vi "EPTx Basic Example FPGA test.vi"() -> ()   [LabVIEW 2019]
uses:
  <vilib>/Powertrain Controls/Device Drivers/Engine Position Tracking/EPTx/RevA/FPGA/Controls/EPTxTooth.ctl
  <vilib>/Powertrain Controls/Device Drivers/Engine Position Tracking/EPTx/RevA/FPGA/Controls/EPTxConfig.ctl
  <vilib>/Powertrain Controls/Device Drivers/Engine Position Tracking/EPTx/RevA/FPGA/Controls/EPTxSupervisor.ctl
  <vilib>/Platform/TimedLoop/XDataNode/timing_clust.ctl
  <vilib>/Platform/TimedLoop/XDataNode/nitl_modes.ctl
  <vilib>/Platform/TimedLoop/XDataNode/wakeup.ctl
  <vilib>/Powertrain Controls/Device Drivers/Engine Position Tracking/EPTx/RevA/FPGA/Controls/EPTxAAPControl.ctl
  <vilib>/Powertrain Controls/Device Drivers/Engine Position Tracking/EPTx/RevA/FPGA/Controls/EPTxSignals.ctl
  <vilib>/Powertrain Controls/Device Drivers/Engine Position Tracking/EPTx/RevA/FPGA/Controls/EPTxControl.ctl
  <vilib>/rvi/Emulation/niFpgaGetClockAttributes.vi
  <vilib>/rvi/Emulation/niFpgaSctlEmulationGetInTimedLoop.vi
  <vilib>/rvi/Emulation/niFpgaEmulationReportErrorSimple.vi
  <vilib>/rvi/eio/common/nirviEmuTemplateMethod_errors.vi
  <vilib>/rvi/Emulation/niFpgaCriticalErrorInLSC.vi
  <vilib>/eio/EIONode/EIONode.xnode
  <vilib>/Platform/TimedLoop/XDataNode/XDataNode.xnode
  <vilib>/Platform/TimedLoop/XDataNode/XDNodeRunTimeDep.lvlib
  <vilib>/Powertrain Controls/Device Drivers/Engine Position Tracking/EPTx/RevA/FPGA/EPTx - RevA - FPGA.lvlib
panel:
  in  "Watchdog":bool
  in  "Sim Rate":fxp<+,24,6> format="%.20g"
  in  "Sim Enable":bool
  in  "Clear Errors":bool
  in  "Sync Enable":bool
  out "Watchdog Error":bool
  out "Aux Warning":bool
  out "Pattern Error":bool
  out "Ratio Error":bool
  out "Overflow":bool
  out "Stall":bool
  out "Rcvg Primary":bool
  out "Config":bool
  out "AvgSpeed":fxp<+,17,15> format="%.7g"
  out "CADRate":fxp<+,22,8> format="%.17g"
  out "HistoryCAD":fxp<+,11,11>
  out "MaxCAD":fxp<+,11,11>
  out "CurrentCAD":fxp<+,18,11> format="%.11g"
  out "Sync":bool
  in  "Cylinder1_L_F [CAD]":fxp<+,18,11> format="%.11g"
  in  "Cylinder1_L_R [CAD]":fxp<+,18,11> format="%.11g"
  in  "Cylinder1_H_F [CAD]":fxp<+,18,11> format="%.11g"
  in  "Cylinder1_H_R [CAD]":fxp<+,18,11> format="%.11g"
  in  "FallingCAD":fxp<+,18,11> format="%.11g"
  in  "RisingCAD":fxp<+,18,11> format="%.11g"
  in  "Enable":bool
  in  "当前转速":fxp<+,24,14>
  out "EPTxSupervisor":T1
  in  "EPTxConfig":T2
  out "EPTxTooth":T3
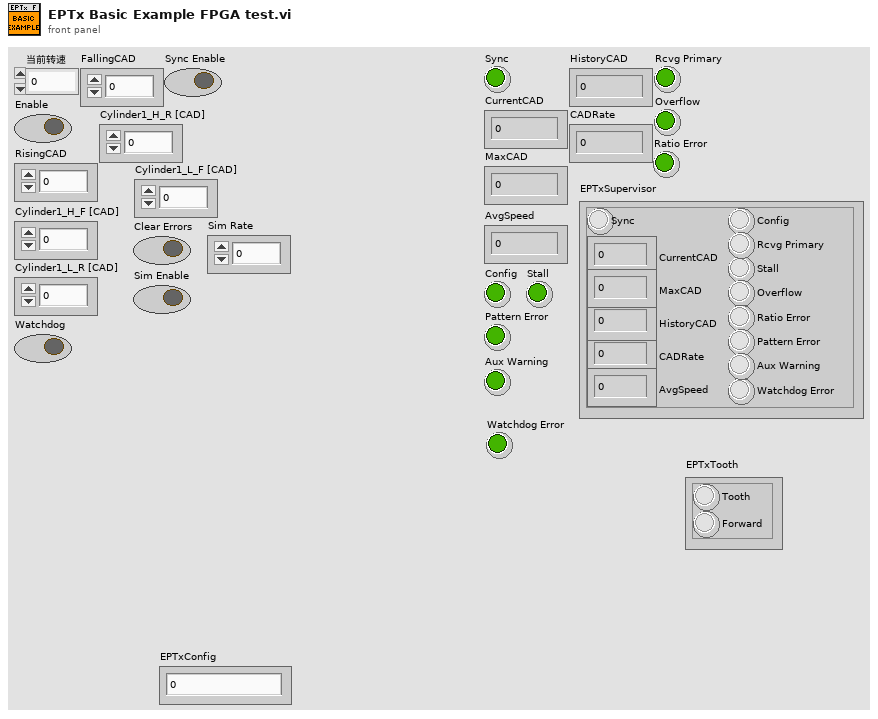
[diagram p1: front panel]
types:
  T1 = typedef "EPTx - RevA - FPGA.lvlib/EPTxSupervisor.ctl" = cluster{"Sync":bool, "CurrentCAD":fxp<+,18,11>, "MaxCAD":fxp<+,11,11>, "HistoryCAD":fxp<+,11,11>, "CADRate":fxp<+,22,8>, "AvgSpeed":fxp<+,17,15>, "Config":bool, "Rcvg Primary":bool, "Stall":bool, "Overflow":bool, "Ratio Error":bool, "Pattern Error":bool, "Aux Warning":bool, "Watchdog Error":bool}
  T2 = typedef "EPTx - RevA - FPGA.lvlib/EPTxConfig.ctl" = u64
  T3 = typedef "EPTx - RevA - FPGA.lvlib/EPTxTooth.ctl" = cluster{"Tooth":bool, "Forward":bool}
  T4 = typedef "XDNodeRunTimeDep.lvlib/timing_clust.ctl" = cluster{"Expected End [f-1]":u64, "Actual End [f-1]":u64, "Finished Late? [f-1]":bool, "Expected End [i-1]":u64, "Actual End [i-1]":u64, "Finished Late? [i-1]":bool, "Expected Start [i]":u64, "Actual Start [i]":u64, "Expected Start [f]":u64, "Actual Start [f]":u64, "Source Name":string, "Structure Name":string, "Period":i64, "Deadline":i64, "Offset":i64, "Start":i64, "Priority":i32, "Timeout":i32, "Mode":T5, "Wakeup Reason":T6, "Error":errorcluster, "Source Type":string, "Secondary Source Type":string, "Global End Time":u64, "Global Start Time":u64, "Frame Duration":u64, "Iteration Duration":u64, "Assigned CPU":i32, "I/O Scan Engine Mode":u32}
  T5 = typedef "XDNodeRunTimeDep.lvlib/nitl_modes.ctl" = enum32{"No Change", "Process missed periods, maintain original phase", "Discard missed periods, maintain original phase", "Process missed periods, ignore original phase", "Discard missed periods, ignore original phase"}
  T6 = typedef "XDNodeRunTimeDep.lvlib/wakeup.ctl" = enum32{"Normal", "Aborted", "Asynchronous wakeup", "Timing source error", "Timed loop error", "Timeout"}
  T7 = typedef "EPTx - RevA - FPGA.lvlib/EPTxControl.ctl" = cluster{"Sync Enable":bool, "Clear Errors":bool, "Sim Enable":bool, "Sim Rate":fxp<+,24,6>, "Watchdog":bool}
  T8 = cluster{"Cylinder1_H_R [CAD]":fxp<+,18,11>, "Cylinder1_H_F [CAD]":fxp<+,18,11>, "Cylinder1_L_R [CAD]":fxp<+,18,11>, "Cylinder1_L_F [CAD]":fxp<+,18,11>}
  T9 = typedef "EPTx - RevA - FPGA.lvlib/EPTxAAPControl.ctl" = cluster{"Enable":bool, "RisingCAD":fxp<+,18,11>, "FallingCAD":fxp<+,18,11>}
  T10 = typedef "EPTx - RevA - FPGA.lvlib/EPTxSignals.ctl" = cluster{"Primary":bool, "Aux 1":bool, "Aux 2":bool, "Aux 3":bool, "Aux 4":bool}
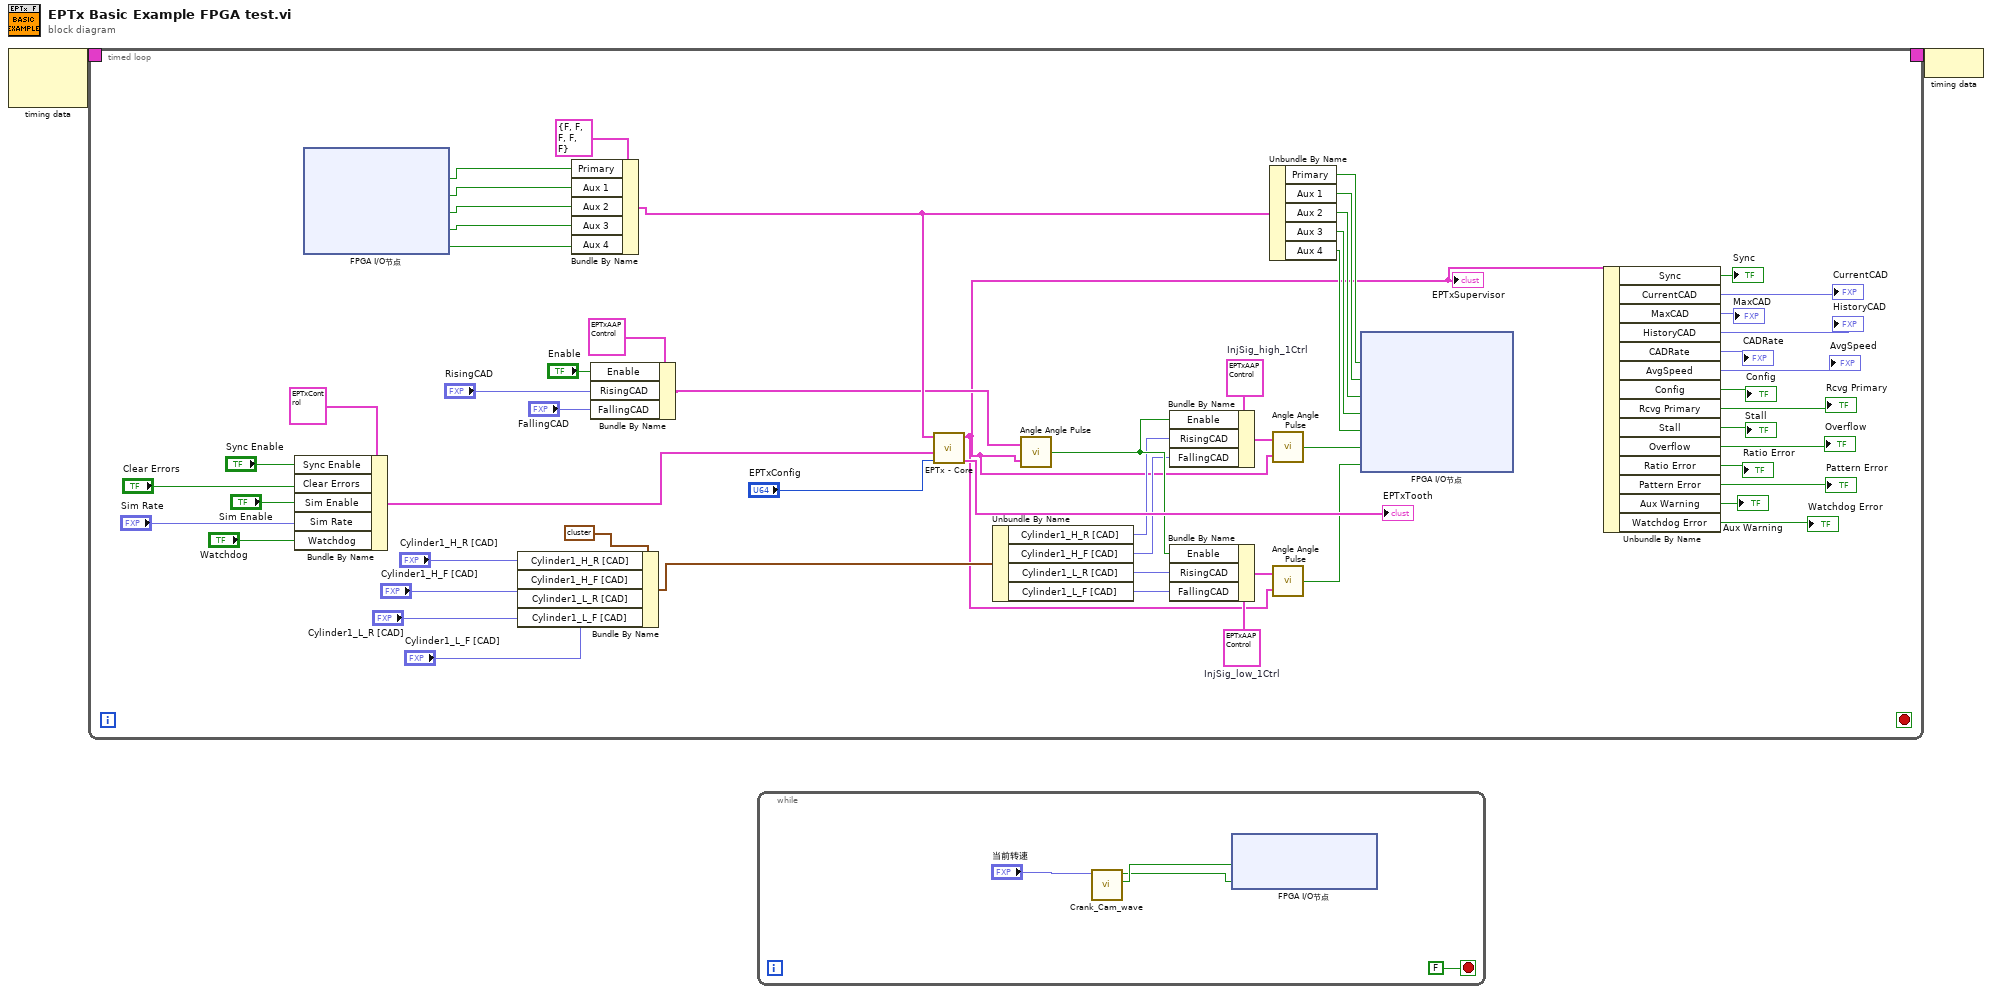
[diagram p0: block diagram]
diagram:
  n1 = node-c288() -> (w2:T4)  [unwired: 2 in]
  n2 = timed-loop {
    timing: w2 -> [_]
    timing-out: [_] -> w1
    stop <- _ stop-if-true
    w51 = T9 {"Enable"=FALSE, "RisingCAD"=0.0, "FallingCAD"=0.0}  # InjSig_low_1Ctrl
    w52 = T9 {"Enable"=FALSE, "RisingCAD"=0.0, "FallingCAD"=0.0}  # InjSig_high_1Ctrl
    n3 = Bundle By Name(cluster=T7 {"Sync Enable"=FALSE, "Clear Errors"=FALSE, "Sim Enable"=FALSE, "Sim Rate"=0.0, "Watchdog"=FALSE} ("EPTxControl"), "Sync Enable"="Sync Enable", "Clear Errors"="Clear Errors", "Sim Enable"="Sim Enable", "Sim Rate"="Sim Rate", "Watchdog"="Watchdog") -> (w3:T7)
    n4 = xnode "FPGA I/O节点"() -> ("Connector1/DIO0"=w40:bool, "Connector1/DIO1"=w39:bool, "Connector1/DIO2"=w38:bool, "Connector1/DIO3"=w37:bool, "Connector1/DIO4"=w36:bool)  [unwired: 5 in, 5 out]
    n5 = Bundle By Name(cluster=T8 {"Cylinder1_H_R [CAD]"=0.0, "Cylinder1_H_F [CAD]"=0.0, "Cylinder1_L_R [CAD]"=0.0, "Cylinder1_L_F [CAD]"=0.0} ("CylinderSig_1"), "Cylinder1_H_R [CAD]"="Cylinder1_H_R [CAD]", "Cylinder1_H_F [CAD]"="Cylinder1_H_F [CAD]", "Cylinder1_L_R [CAD]"="Cylinder1_L_R [CAD]", "Cylinder1_L_F [CAD]"="Cylinder1_L_F [CAD]") -> (w25:T8)
    n6 = Bundle By Name(cluster=T10 {"Primary"=FALSE, "Aux 1"=FALSE, "Aux 2"=FALSE, "Aux 3"=FALSE, "Aux 4"=FALSE} ("EPTxSignals"), "Primary"=w40, "Aux 1"=w39, "Aux 2"=w38, "Aux 3"=w37, "Aux 4"=w36) -> (w41:T10)
    n7 = Bundle By Name(cluster=T9 {"Enable"=FALSE, "RisingCAD"=0.0, "FallingCAD"=0.0} ("AAPControl_1str"), "Enable"="Enable", "RisingCAD"="RisingCAD", "FallingCAD"="FallingCAD") -> (w31:T9)
    n8 = call <vilib>:"EPTx - Core.vi"("EPTxConfig"="EPTxConfig", "EPTxControl"=w3, "EPTxSignals"=w41) -> ("EPTxTooth"=→"EPTxTooth":T3, "EPTxSupervisor"=w24:T1)  [unwired: 7 in]
    "EPTxSupervisor" <- w24
    n9 = Unbundle By Name(w25) -> ("Cylinder1_H_R [CAD]"=w48:fxp<+,18,11>, "Cylinder1_H_F [CAD]"=w47:fxp<+,18,11>, "Cylinder1_L_R [CAD]"=w46:fxp<+,18,11>, "Cylinder1_L_F [CAD]"=w45:fxp<+,18,11>)
    n10 = call <vilib>:"Angle Angle Pulse.vi"("EPTxSupervisor"=w24, "AAPControl"=w31) -> ("AAP"=w49:bool)
    n11 = Bundle By Name(cluster=w52, "Enable"=w49, "RisingCAD"=w48, "FallingCAD"=w47) -> (w53:T9)
    n12 = Bundle By Name(cluster=w51, "Enable"=w49, "RisingCAD"=w46, "FallingCAD"=w45) -> (w50:T9)
    n13 = Unbundle By Name(w41) -> ("Primary"=w58:bool, "Aux 1"=w57:bool, "Aux 2"=w56:bool, "Aux 3"=w55:bool, "Aux 4"=w54:bool)
    n14 = call <vilib>:"Angle Angle Pulse.vi"("EPTxSupervisor"=w24, "AAPControl"=w53) -> ("AAP"=w44:bool)
    n15 = call <vilib>:"Angle Angle Pulse.vi"("EPTxSupervisor"=w24, "AAPControl"=w50) -> ("AAP"=w43:bool)
    n16 = xnode "FPGA I/O节点"("Connector0/DIO4"=w58, "Connector0/DIO5"=w57, "Connector0/DIO6"=w56, "Connector0/DIO7"=w55, "Connector0/DIO8"=w54, "Connector0/DIO9"=w44, "Connector0/DIO10"=w43) -> ()  [unwired: 7 in, 7 out]
    n17 = Unbundle By Name(w24) -> ("Sync"=→"Sync":bool, "CurrentCAD"=→"CurrentCAD":fxp<+,18,11>, "MaxCAD"=→"MaxCAD":fxp<+,11,11>, "HistoryCAD"=→"HistoryCAD":fxp<+,11,11>, "CADRate"=→"CADRate":fxp<+,22,8>, "AvgSpeed"=→"AvgSpeed":fxp<+,17,15>, "Config"=→"Config":bool, "Rcvg Primary"=→"Rcvg Primary":bool, "Stall"=→"Stall":bool, "Overflow"=→"Overflow":bool, "Ratio Error"=→"Ratio Error":bool, "Pattern Error"=→"Pattern Error":bool, "Aux Warning"=→"Aux Warning":bool, "Watchdog Error"=→"Watchdog Error":bool)
  }
  n18 = while {
    stop <- FALSE stop-if-true
    n19 = call "Crank_Cam_wave.vi"("当前转速"="当前转速") -> ("曲轴"=w64:bool, "凸轮轴"=w63:bool)  [unwired: 9 in]
    n20 = xnode "FPGA I/O节点"("Connector0/DIO0"=w64, "Connector0/DIO1"=w63) -> ()  [unwired: 2 in, 2 out]
  }
  n21 = node-c288(w1) -> ()
